vi "MGCC_FntStaMach_Initial_flag.vi"   [LabVIEW 2016]
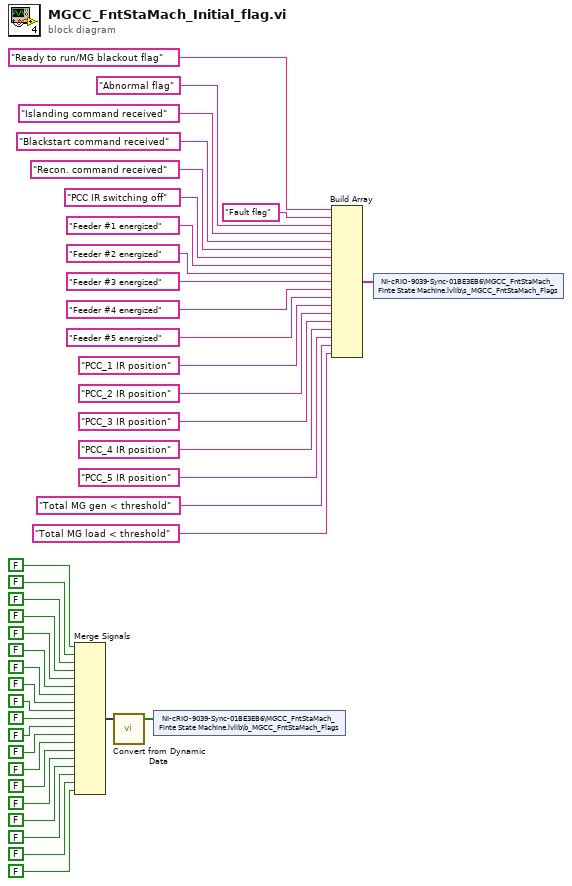
[diagram p0: block diagram]
diagram:
  n1 = Merge Signals(FALSE ("State3"), FALSE ("State3"), FALSE ("State3"), FALSE ("State3"), FALSE ("State3"), FALSE ("State3"), FALSE ("State3"), FALSE ("State3"), FALSE ("State3"), FALSE ("State3"), FALSE ("State3"), FALSE ("State3"), FALSE ("State3"), FALSE ("State3"), FALSE ("State3"), FALSE ("State3"), FALSE ("State3"), FALSE ("State3"), FALSE ("State3")) -> (w31:dynamicdata)
  n2 = call "Convert from Dynamic Data"("Dynamic Data Type"=w31) -> ("Array"=w19:bool[])  [unwired: 3 in]
  n3 = shared-variable "NI-cRIO-9039-Sync-01BE3EB6\\MGCC_FntStaMach_Finte State Machine.lvlib\\b_MGCC_FntStaMach_Flags"(w19) -> ()  [unwired: 1 in, 1 out]
  n4 = Build Array("Ready to run/MG blackout flag", "Fault flag", "Abnormal flag", "Islanding command received", "Blackstart command received", "Recon. command received", "PCC IR switching off", "Feeder #1 energized", "Feeder #2 energized", "Feeder #3 energized", "Feeder #4 energized", "Feeder #5 energized", "PCC_1 IR position", "PCC_2 IR position", "PCC_3 IR position", "PCC_4 IR position", "PCC_5 IR position", "Total MG gen < threshold", "Total MG load < threshold") -> (w20:string[])
  n5 = shared-variable "NI-cRIO-9039-Sync-01BE3EB6\\MGCC_FntStaMach_Finte State Machine.lvlib\\s_MGCC_FntStaMach_Flags"(w20) -> ()  [unwired: 1 in, 1 out]
